vi "Assign DRC values.vi"(2 "Queried Rec. table":i32[](array[numeric]), 4 "Input String":string, 5 "error in":errorcluster) -> (14 "Rec. option":i32[](array[numeric]), 15 "Source ID":string[](array[string]), 16 "Trigger option":i32[](array[numeric]), 17 "Queried Rec. table out":i32[](array[numeric]), 18 "Rec. option string":string[](array[string]), 19 "error out":errorcluster)   [LabVIEW 2026]
doc: "This VI assigns values (Source ID and Rec. option) from input string to queried Rec. tables. Sub-VI for DRC?.vi.\nGCS 2.0: Trigger option is not valid."
panel:
  # "This vi assigns values (Source ID, Rec. option, Trigger option) from input string to queried Rec. tables"
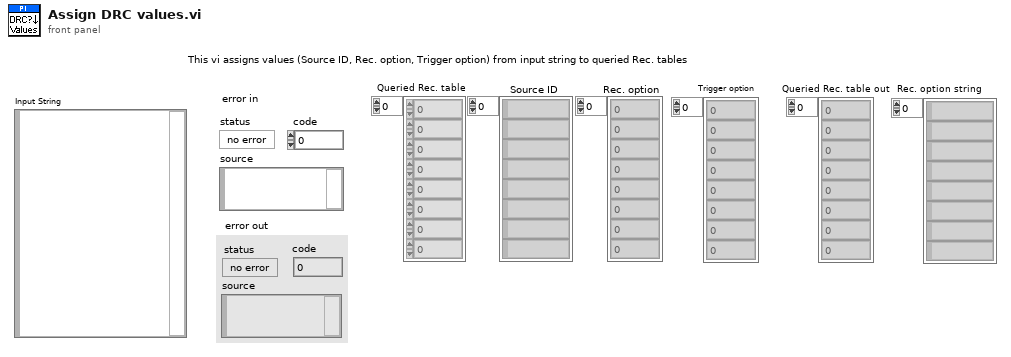
[diagram p1: front panel]
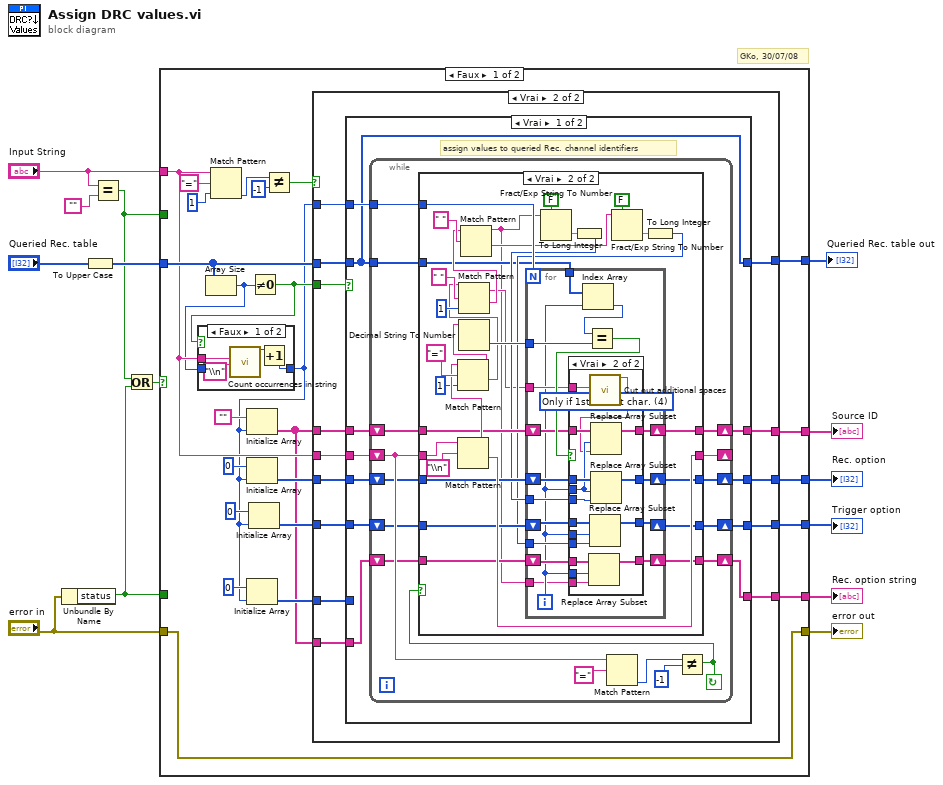
[diagram p0: block diagram]
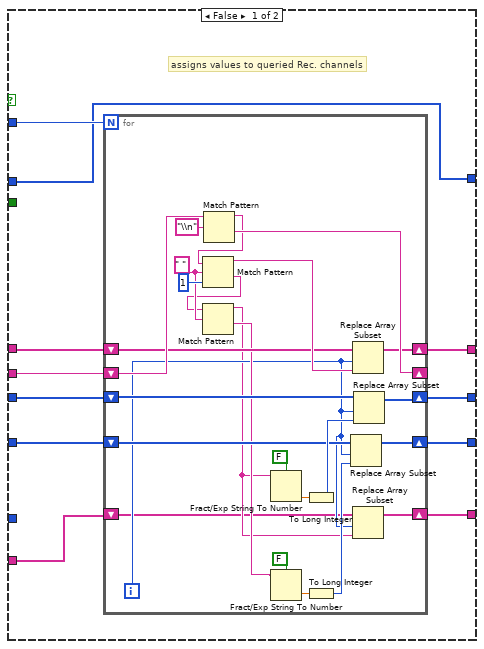
[diagram p3: hidden frame]
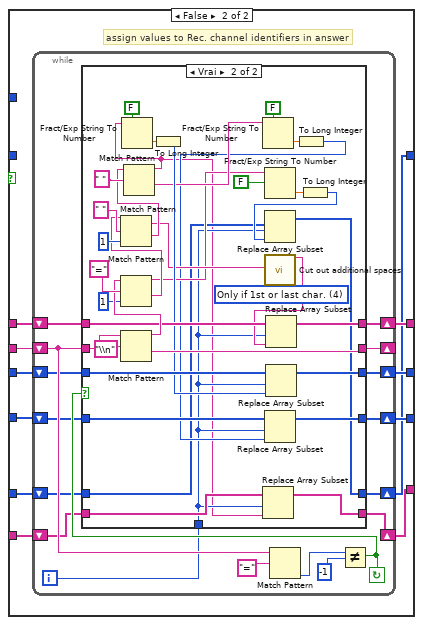
[diagram p6: hidden frame]
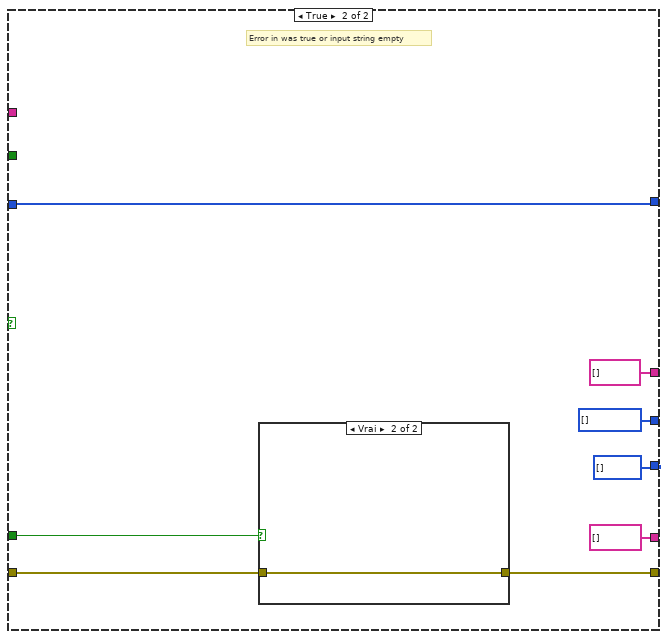
[diagram p8: hidden frame]
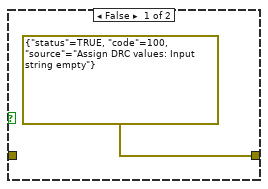
[diagram p9: hidden frame]
diagram:
  # "GKo, 30/07/08"
  n1 = Unbundle By Name("error in") -> ("status"=w5:bool)
  n2 = To Upper Case(1:"Queried Rec. table") -> (0:w7:i32[])
  n3 = Equal?(x="Input String", y="") -> (x = y?=w4:bool)
  n4 = Or(x=w4, y=w5) -> (x .or. y?=w8:bool)
  n5 = case shown="Faux" w8 {
    tunnel: "Input String" -> [w23 _]
    tunnel: [w38 i32[] [] ("Step Size")] -> w14
    tunnel: w7 -> [w37 w268]
    tunnel: [w36 w272] -> w11
    tunnel: "error in" -> [w36 w273]
    tunnel: w4 -> [_ _]
    tunnel: [w35 string[] []] -> w6
    tunnel: w5 -> [_ w270]
    tunnel: [w26 i32[] []] -> w3
    tunnel: [w20 w268] -> w2
    tunnel: [w15 string[] []] -> w1
    frame False {
      n6 = Array Size(array=w37) -> (size(s)=w22:i32)
      n7 = Match Pattern(string=w23, regular expression="=", offset (0)=1) -> (offset past match=w32:i32)  [unwired: 3 out]
      n8 = Not Equal To 0?(x=w22) -> (x != 0?=w21:bool)
      n9 = case shown="Faux" w21 {
        tunnel: [w39 w43] -> w17
        tunnel: w22 -> [_ w43]
        tunnel: w23 -> [w42 _]
        frame False {
          n10 = call "Count occurrences in string.vi"("Input string"=w42, "Expression"="\\n") -> ("Occurrences"=w40:i32)  [unwired: 17 out]
          n11 = Increment(x=w40) -> (x+1=w39:i32)
        }
        frame True {
        }
      }
      n12 = Initialize Array("", w17) -> (w16:string[])
      n13 = Initialize Array(0 ("Element Data"), w17) -> (w29:i32[])
      n14 = Initialize Array(0 ("Element Data"), w17) -> (w18:i32[])
      n15 = Initialize Array(0 ("Element Data"), w17) -> (w24:i32[])
      n16 = Not Equal?(x=w32, y=-1) -> (x != y?=w31:bool)
      n17 = case shown="Vrai" w31 {
        tunnel: [w54 w92] -> w38
        tunnel: w23 -> [w53 w93]
        tunnel: w37 -> [w46 w91]
        tunnel: w29 -> [w52 w89]
        tunnel: w17 -> [w51 w90]
        tunnel: w16 -> [w50 w88]
        tunnel: [w49 w87] -> w35
        tunnel: [w48 w85] -> w26
        tunnel: w24 -> [w47 w86]
        tunnel: w21 -> [_ w84]
        tunnel: [w46 w83] -> w20
        tunnel: w18 -> [_ w82]
        tunnel: w16 -> [w44 w81]
        tunnel: [w45 w80] -> w15
        frame False {
          # "assigns values to queried Rec. channels"
          n18 = for {
            N: w51 -> [_]
            shift-right: [w68] -> w54
            shift-left: w52 -> [w69]
            shift-right: [w78] -> _
            shift-left: w53 -> [w79]
            shift-right: [w71] -> w49
            shift-left: w50 -> [w72]
            shift-right: [w61] -> w48
            shift-left: w47 -> [w60]
            shift-right: [w58] -> w45
            shift-left: w44 -> [w55]
            i -> [w57]
            w67 = " " ("regular expression")
            n19 = Match Pattern(string=w79, regular expression="\\n") -> (before substring=w74:string, after substring=w78:string)  [unwired: 3 out]
            n20 = Match Pattern(string=w74, regular expression=w67, offset (0)=1) -> (before substring=w73:string, after substring=w66:string)  [unwired: 2 out]
            n21 = Match Pattern(string=w66, regular expression=w67) -> (before substring=w56:string, after substring=w59:string)  [unwired: 3 out]
            n22 = Fract/Exp String To Number(use system decimal point (T)=FALSE, string=w56) -> (number=w75:dbl)  [unwired: 3 out]
            n23 = Fract/Exp String To Number(use system decimal point (T)=FALSE, string=w59) -> (number=w64:dbl)  [unwired: 3 out]
            n24 = To Long Integer(number=w75) -> (32bit integer=w70:i32)
            n25 = To Long Integer(number=w64) -> (32bit integer=w62:i32)
            n26 = Replace Array Subset(array=w60, new element=w62, index=w57) -> (w61:i32[])
            n27 = Replace Array Subset(array=w72, new element=w73, index=w57) -> (w71:string[])
            n28 = Replace Array Subset(array=w55, new element=w56, index=w57) -> (w58:string[])
            n29 = Replace Array Subset(array=w69, new element=w70, index=w57) -> (w68:i32[])
          }
        }
        frame True {
          n30 = case shown="Vrai" w84 {
            tunnel: w93 -> [w104 w206]
            tunnel: [w103 w205] -> w92
            tunnel: w91 -> [w96 _]
            tunnel: w90 -> [w102 _]
            tunnel: w89 -> [w101 w204]
            tunnel: w88 -> [w100 w203]
            tunnel: [w99 w202] -> w87
            tunnel: w86 -> [w98 w201]
            tunnel: [w97 w200] -> w85
            tunnel: [w96 w198] -> w83
            tunnel: w82 -> [_ w199]
            tunnel: w81 -> [w95 w197]
            tunnel: [w94 w196] -> w80
            frame True {
              # "assign values to queried Rec. channel identifiers"
              n31 = while {
                shift-left: w98 -> [w107]
                shift-right: [w108] -> w97
                shift-left: w100 -> [w109]
                shift-right: [w110] -> w99
                tunnel: w102 -> [w111]
                tunnel: w96 -> [w112]
                shift-left: w101 -> [w114]
                shift-right: [w113] -> w103
                shift-left: w104 -> [w117]
                shift-right: [w116] -> _
                shift-right: [w105] -> w94
                shift-left: w95 -> [w106]
                stop <- w115 continue-if-true
                n32 = Match Pattern(string=w117, regular expression="=") -> (offset past match=w118:i32)  [unwired: 4 out]
                n33 = Not Equal?(x=w118, y=-1) -> (x != y?=w115:bool)
                n34 = case shown="Vrai" w115 {
                  tunnel: w117 -> [w125 w156]
                  tunnel: [w125 w155] -> w116
                  tunnel: [w124 w153] -> w113
                  tunnel: w114 -> [w124 w154]
                  tunnel: w112 -> [_ w130]
                  tunnel: w111 -> [_ w150]
                  tunnel: [w123 w149] -> w110
                  tunnel: w109 -> [w123 w148]
                  tunnel: [w122 w134] -> w108
                  tunnel: w107 -> [w122 w133]
                  tunnel: w106 -> [w121 w129]
                  tunnel: [w121 w128] -> w105
                  frame False {
                  }
                  frame True {
                    n35 = Match Pattern(string=w156, regular expression="\\n") -> (before substring=w151:string, after substring=w155:string)  [unwired: 3 out]
                    n36 = Match Pattern(string=w151, regular expression="=", offset (0)=1) -> (before substring=w146:string, after substring=w141:string)  [unwired: 2 out]
                    n37 = Match Pattern(string=w141, regular expression=" ", offset (0)=1) -> (before substring=w131:string, after substring=w137:string)  [unwired: 2 out]
                    n38 = Decimal String To Number(string=w146) -> (number=w145:i32)  [unwired: 3 out]
                    n39 = Match Pattern(string=w137, regular expression=" ") -> (before substring=w126:string, after substring=w127:string)  [unwired: 3 out]
                    n40 = Fract/Exp String To Number(use system decimal point (T)=FALSE, string=w126) -> (number=w140:dbl)  [unwired: 3 out]
                    n41 = To Long Integer(number=w140) -> (32bit integer=w139:i32)
                    n42 = Fract/Exp String To Number(use system decimal point (T)=FALSE, string=w127) -> (number=w135:dbl)  [unwired: 3 out]
                    n43 = To Long Integer(number=w135) -> (32bit integer=w132:i32)
                    n44 = for {
                      N: w150 -> [_]
                      tunnel: w139 -> [w174]
                      shift-right: [w172] -> w153
                      shift-left: w154 -> [w173]
                      tunnel: w145 -> [w170]
                      shift-right: [w167] -> w149
                      shift-left: w148 -> [w168]
                      tunnel: w131 -> [w166]
                      tunnel: w130 -> [w165]
                      shift-right: [w164] -> w134
                      shift-left: w133 -> [w163]
                      tunnel: w132 -> [w162]
                      shift-right: [w161] -> w128
                      shift-left: w129 -> [w160]
                      tunnel: w126 -> [w158]
                      i -> [w159]
                      n45 = Index Array(array=w165, index=w159) -> (element=w171:i32)
                      n46 = Equal?(x=w171, y=w170) -> (x = y?=w169:bool)
                      n47 = case shown="Vrai" w169 {
                        tunnel: w174 -> [_ w195]
                        tunnel: w159 -> [_ w192]
                        tunnel: w173 -> [w178 w194]
                        tunnel: [w178 w193] -> w172
                        tunnel: w168 -> [w177 w191]
                        tunnel: [w177 w190] -> w167
                        tunnel: w166 -> [_ w184]
                        tunnel: [w176 w189] -> w164
                        tunnel: w163 -> [w176 w188]
                        tunnel: w159 -> [_ w187]
                        tunnel: w162 -> [_ w186]
                        tunnel: [w175 w182] -> w161
                        tunnel: w160 -> [w175 w181]
                        tunnel: w159 -> [_ w180]
                        tunnel: w158 -> [_ w179]
                        frame False {
                        }
                        frame True {
                          w185 = u16 4 items=["All Spaces", "Only if 1st char.", "Only if last char.", "Only if near \"=\"", "Only if 1st or last char.", "Only multiple"] ("Mode")
                          n48 = Replace Array Subset(array=w181, new element=w179, index=w180) -> (w182:string[])
                          n49 = call "Cut out additional spaces.vi"("String"=w184, "Mode"=w185) -> ("String out"=w183:string)  [unwired: 17 out]
                          n50 = Replace Array Subset(array=w188, new element=w186, index=w187) -> (w189:i32[])
                          n51 = Replace Array Subset(array=w191, new element=w183, index=w192) -> (w190:string[])
                          n52 = Replace Array Subset(array=w194, new element=w195, index=w192) -> (w193:i32[])
                        }
                      }
                    }
                  }
                }
              }
            }
            frame False {
              # "assign values to Rec. channel identifiers in answer"
              n53 = while {
                shift-left: w201 -> [w212]
                shift-right: [w213] -> w200
                shift-left: w203 -> [w214]
                shift-right: [w215] -> w202
                shift-left: w204 -> [w217]
                shift-right: [w216] -> w205
                shift-left: w206 -> [w220]
                shift-right: [w219] -> _
                shift-right: [w210] -> w198
                shift-left: w199 -> [w211]
                shift-right: [w207] -> w196
                shift-left: w197 -> [w208]
                i -> [w209]
                stop <- w218 continue-if-true
                n54 = Match Pattern(string=w220, regular expression="=") -> (offset past match=w221:i32)  [unwired: 4 out]
                n55 = Not Equal?(x=w221, y=-1) -> (x != y?=w218:bool)
                n56 = case shown="Vrai" w218 {
                  tunnel: w220 -> [w229 w265]
                  tunnel: [w229 w264] -> w219
                  tunnel: [w228 w262] -> w216
                  tunnel: w217 -> [w228 w263]
                  tunnel: [w227 w259] -> w215
                  tunnel: w214 -> [w227 w258]
                  tunnel: [w226 w245] -> w213
                  tunnel: w212 -> [w226 w244]
                  tunnel: w211 -> [w225 w235]
                  tunnel: [w225 w234] -> w210
                  tunnel: w209 -> [_ w232]
                  tunnel: w208 -> [w224 w233]
                  tunnel: [w224 w230] -> w207
                  frame False {
                  }
                  frame True {
                    w242 = u16 4 items=["All Spaces", "Only if 1st char.", "Only if last char.", "Only if near \"=\"", "Only if 1st or last char.", "Only multiple"] ("Mode")
                    n57 = Match Pattern(string=w265, regular expression="\\n") -> (before substring=w260:string, after substring=w264:string)  [unwired: 3 out]
                    n58 = Match Pattern(string=w260, regular expression="=", offset (0)=1) -> (before substring=w238:string, after substring=w253:string)  [unwired: 2 out]
                    n59 = Match Pattern(string=w253, regular expression=" ", offset (0)=1) -> (before substring=w243:string, after substring=w249:string)  [unwired: 2 out]
                    n60 = Match Pattern(string=w249, regular expression=" ") -> (before substring=w231:string, after substring=w246:string)  [unwired: 3 out]
                    n61 = Fract/Exp String To Number(use system decimal point (T)=FALSE, string=w231) -> (number=w252:dbl)  [unwired: 3 out]
                    n62 = To Long Integer(number=w252) -> (32bit integer=w251:i32)
                    n63 = Fract/Exp String To Number(use system decimal point (T)=FALSE, string=w246) -> (number=w247:dbl)  [unwired: 3 out]
                    n64 = Replace Array Subset(array=w233, new element=w231, index=w232) -> (w230:string[])
                    n65 = Fract/Exp String To Number(use system decimal point (T)=FALSE, string=w238) -> (number=w239:dbl)  [unwired: 3 out]
                    n66 = call "Cut out additional spaces.vi"("String"=w243, "Mode"=w242) -> ("String out"=w241:string)  [unwired: 17 out]
                    n67 = Replace Array Subset(array=w258, new element=w241, index=w232) -> (w259:string[])
                    n68 = Replace Array Subset(array=w263, new element=w251, index=w232) -> (w262:i32[])
                    n69 = To Long Integer(number=w247) -> (32bit integer=w237:i32)
                    n70 = Replace Array Subset(array=w244, new element=w237, index=w232) -> (w245:i32[])
                    n71 = To Long Integer(number=w239) -> (32bit integer=w236:i32)
                    n72 = Replace Array Subset(array=w235, new element=w236, index=w232) -> (w234:i32[])
                  }
                }
              }
            }
          }
        }
      }
    }
    frame True {
      # "Error in was true or input string empty"
      n73 = case shown="Vrai" w270 {
        tunnel: w273 -> [_ w276]
        tunnel: [errorcluster {"status"=TRUE, "code"=100, "source"="Assign DRC values: Input string empty"} ("error out") w276] -> w272
        frame False {
        }
        frame True {
        }
      }
    }
  }
  "Rec. option" <- w14
  "error out" <- w11
  "Source ID" <- w6
  "Trigger option" <- w3
  "Queried Rec. table out" <- w2
  "Rec. option string" <- w1
